vi "Beep and Blink.vi"() -> ()   [LabVIEW 2018]
uses:
  EPU452 Class/EPU452.lvclass
panel:
  in  "BEEP":bool
  in  "Stop":bool
  in  "COM Port":refnum<visa-resource-name>
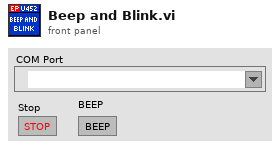
[diagram p1: front panel]
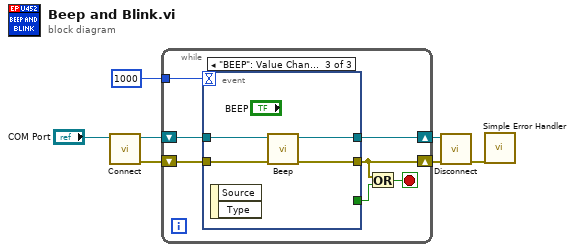
[diagram p0: block diagram]
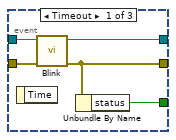
[diagram p2: hidden frame]
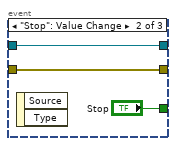
[diagram p3: hidden frame]
diagram:
  n1 = call "Connect.vi"("COM Port"="COM Port") -> ("error out"=w3:errorcluster, "EPU452 out"=w4:refnum<class "EPU452.lvclass">)  [unwired: 9 in]
  n2 = while {
    tunnel: 1000 -> [w14]
    shift-right: [w11] -> w2
    shift-left: w4 -> [w13]
    shift-right: [w9] -> w1
    shift-left: w3 -> [w12]
    stop <- w8 stop-if-true
    n3 = event shown="[2] \"BEEP\": Value Change" {
      selector: _ -> [_ _ _]
      dyn-events: _ -> [_ _ _]
      timeout: w14 -> [_ _ _]
      tunnel: [w15 "Stop" _] -> w10
      tunnel: w13 -> [w19 w20 w26]
      tunnel: w12 -> [w18 w21 w25]
      tunnel: [w16 w21 w23] -> w9
      tunnel: [w17 w20 w24] -> w11
      event Timeout {
        n4 = event-data() -> ()  [unwired: 1 in, 1 out]
        n5 = call "Blink.vi"("error in (no error)"=w18, "EPU452 in"=w19) -> ("error out"=w16:errorcluster, "EPU452 out"=w17:refnum<class "EPU452.lvclass">)  [unwired: 8 in]
        n6 = Unbundle By Name(w16) -> ("status"=w15:bool)
      }
      event "Stop": Value Change {
        n7 = event-data() -> ()  [unwired: 1 in, 2 out]
      }
      event "BEEP": Value Change {
        n8 = event-data() -> ()  [unwired: 1 in, 2 out]
        n9 = call "Beep.vi"("error in (no error)"=w25, "EPU452 in"=w26) -> ("error out"=w23:errorcluster, "EPU452 out"=w24:refnum<class "EPU452.lvclass">)  [unwired: 8 in]
      }
    }
    n10 = Or(x=w9, y=w10) -> (x .or. y?=w8:bool)
  }
  n11 = call "Disconnect.vi"("error in (no error)"=w1, "EPU452 in"=w2) -> ("error out"=w7:errorcluster)  [unwired: 9 in]
  n12 = call <vilib>:"Simple Error Handler.vi"("error in (no error)"=w7) -> ()  [unwired: 4 in, 5 out]
